vi "main(Test DQMH modules).bak.vi"() -> ()   [LabVIEW 2018, in "Application.lvlib"] (continued)
            frame 0 {
              n828 = Initialize Array(FALSE, 6 ("dimension size")) -> (w2002:bool[])
              n829 = call "MB01_eMICs.vi"("Array"=w2002) -> ("error out"=w2005:errorcluster)  [unwired: 10 in]
            }
            frame 1 {
              n830 = call "demux1-10_chan0.vi"() -> ("error out"=w2006:errorcluster)  [unwired: 11 in]
            }
            frame 2 {
              n831 = call "SC enable OFF.vi"() -> ("error out"=w2007:errorcluster)  [unwired: 11 in]
            }
            frame 3 {
              n832 = call "mux10-1_chan0.vi"() -> ("error out"=w2008:errorcluster)  [unwired: 11 in]
            }
            frame 4 {
              n833 = call "mux6-1_chan0.vi"() -> ("error out"=w2009:errorcluster)  [unwired: 11 in]
            }
            frame 5.., Default {
            }
          }
          n834 = Wait (ms)(milliseconds to wait=u32 70) -> ()  [unwired: 1 out]
        }
        n835 = Merge Errors(w1985, w1989) -> (w1982:errorcluster)
      }
      frame "MEAS.AllRelaysOFF2" {
        n836 = disable-structure shown="LOGGING==TRUE" {
          disable-tunnel: w2013 -> [w2027 _]
          frame condition #0 (active) {
            n837 = Empty String/Path?(string/path=w2027) -> (empty?=w2030:bool)
            n838 = Select(t="Quece timeout", s=w2030, f=w2027) -> (s? t:f=w2026:string)
            n839 = call "string log (SubVI).vi"("Enum"=enum16{"Init", "Log", "Read"}."Log", "state Name"=w2026) -> ()  [unwired: 8 in, 2 out]
          }
          frame condition #1 {
          }
        }
        n840 = flat-sequence {
          tunnel: [w2025] -> w2011
          frame #0 {
            n841 = Initialize Array(FALSE, 6 ("dimension size")) -> (w2024:bool[])
            n842 = call "MB01_eMICs.vi"("Array"=w2024) -> ("error out"=w2025:errorcluster)  [unwired: 10 in]
            n843 = Wait (ms)(milliseconds to wait=u32 70) -> ()  [unwired: 1 out]
          }
        }
        n844 = Merge Errors(w2014, w2011) -> (w2010:errorcluster)
      }
      frame "MEAS.Read TRIGGER" {
        w2042 = T10 {"new board?"=TRUE, "new trigger"=TRUE, "last trigger"=TRUE}  # trigger infor
        # "JIG locked - rising-edge happens"
        n845 = disable-structure shown="LOGGING==TRUE" {
          disable-tunnel: w2046 -> [w2060 _]
          frame condition #0 (active) {
            n846 = Empty String/Path?(string/path=w2060) -> (empty?=w2063:bool)
            n847 = Select(t="Quece timeout", s=w2063, f=w2060) -> (s? t:f=w2059:string)
            n848 = call "string log (SubVI).vi"("Enum"=enum16{"Init", "Log", "Read"}."Log", "state Name"=w2059) -> ()  [unwired: 8 in, 2 out]
          }
          frame condition #1 {
          }
        }
        n849 = call "Read JIG trigger.vi"() -> ("error out"=w2050:errorcluster, "Trigger?"=w2032:bool)  [unwired: 9 in, 1 out]
        "trigger Value" <- w2032
        n850 = feedback-in #3(w2032) -> ()
        n851 = feedback #3(FALSE) -> (w2039:bool)
        n852 = Greater?(x=w2032, y=w2039) -> (0:w2034:bool)
        n853 = Bundle By Name(cluster=w2042, "new board?"=w2034, "new trigger"=w2032, "last trigger"=w2039) -> (w2041:T10)
        n854 = local read "Auto/Man"() -> (w2031:bool)
        n855 = Select(t=-1, s=w2034, f=w2036) -> (s? t:f=w2037:i32)
        n856 = local write "New board?"(w2034) -> ()
        n857 = local write "new Trigger?"(w2032) -> ()
        n858 = local write "last Trigger?"(w2039) -> ()
        n859 = And(x=w2031, y=w2034) -> (x .and. y?=w2033:bool)
        n860 = Merge Errors(w2049, w2050) -> (w2047:errorcluster)
        n861 = case shown="True" w2033 {
          tunnel: w2043 -> [_ w2058]
          tunnel: w2041 -> [_ w2057]
          tunnel: [_ w2056] -> w2040
          frame False {
          }
          frame True {
            n862 = Generate User Event(user event=w2058, event data cluster=w2057) -> (error out=w2056:errorcluster)  [unwired: 2 in, 1 out]
          }
        }
        n863 = Merge Errors(w2047, w2040) -> (w2044:errorcluster)
        n864 = flat-sequence {
          tunnel: [w2064] -> w2048
          tunnel: w2044 -> [w2064]
          frame #0 {
            n865 = Wait (ms)(milliseconds to wait=u32 10) -> ()  [unwired: 1 out]
          }
        }
      }
      frame "MEAS.Sel Input Current" {
        n866 = disable-structure shown="LOGGING==TRUE" {
          disable-tunnel: w2067 -> [w2082 _]
          frame condition #0 (active) {
            n867 = Empty String/Path?(string/path=w2082) -> (empty?=w2085:bool)
            n868 = Select(t="Quece timeout", s=w2085, f=w2082) -> (s? t:f=w2081:string)
            n869 = call "string log (SubVI).vi"("Enum"=enum16{"Init", "Log", "Read"}."Log", "state Name"=w2081) -> ()  [unwired: 8 in, 2 out]
          }
          frame condition #1 {
          }
        }
        n870 = Variant To Data(type=enum16{"DMM I (0.5)", "DMM I (12)"}."DMM I (0.5)" ("mux2-1(DMM I) encode"), Variant=w2075) -> (data=w2074:enum16{"DMM I (0.5)", "DMM I (12)"})  [unwired: 1 in, 1 out]
        n871 = call "DMM I 0.5_10.vi"("mux2-1(DMM I) encode"=w2074) -> ("error out"=w2077:errorcluster)  [unwired: 10 in]
        n872 = Merge Errors(w2070, w2077) -> (w2068:errorcluster)
        n873 = flat-sequence {
          tunnel: [w2086] -> w2069
          tunnel: w2068 -> [w2086]
          frame #0 {
            n874 = Wait (ms)(milliseconds to wait=u32 70) -> ()  [unwired: 1 out]
          }
        }
      }
      frame "MEAS.Read Optos" {
        n875 = disable-structure shown="LOGGING==TRUE" {
          disable-tunnel: w2091 -> [w2116 _]
          frame condition #0 (active) {
            n876 = Empty String/Path?(string/path=w2116) -> (empty?=w2119:bool)
            n877 = Select(t="Quece timeout", s=w2119, f=w2116) -> (s? t:f=w2115:string)
            n878 = call "string log (SubVI).vi"("Enum"=enum16{"Init", "Log", "Read"}."Log", "state Name"=w2115) -> ()  [unwired: 8 in, 2 out]
          }
          frame condition #1 {
          }
        }
        n879 = flat-sequence {
          tunnel: [w2105] -> w2089
          frame #0 {
            n880 = disable-structure shown="Enabled" {
              frame Enabled {
                n881 = Wait (ms)(milliseconds to wait=u32 100) -> ()  [unwired: 1 out]
              }
              frame Disabled {
              }
            }
            n882 = Initialize Array(FALSE, 6 ("dimension size"), 10 ("dimension size")) -> (w2100:bool[][])
            n883 = local write "Short DRV"(w2100) -> ()
          }
          frame #1 {
            n884 = call "inst.Optos.vi"() -> ("error out"=w2114:errorcluster, "Optos"=w2112:bool[])  [unwired: 9 in, 1 out]
            n885 = Reshape Array(w2112, 10 ("dimension size"), 6 ("dimension size")) -> (w2110:bool[][])
            n886 = To Variant(anything=w2112) -> (Variant=w2113:variant)
            n887 = Transpose 2D Array(2D array=w2110) -> (transposed array=→"Short DRV":bool[][])
            n888 = call "FGV Driver Data.vi"("Mode"=DUT_data_Mode."Short Circuits", "error in (no error)"=w2114, "FGV enum(Read)"=FGV_DRV_data."Write" ("FGV DRV data enum"), "data"=w2113) -> ("error out"=w2105:errorcluster)  [unwired: 4 in, 3 out]
          }
        }
        n889 = Merge Errors(w2090, w2089) -> (w2092:errorcluster)
        n890 = flat-sequence {
          tunnel: [w2120] -> w2093
          tunnel: w2092 -> [w2120]
          frame #0 {
            n891 = Wait (ms)(milliseconds to wait=u32 70) -> ()  [unwired: 1 out]
          }
        }
      }
      frame "MEAS.Reset JIG" {
        n892 = disable-structure shown="LOGGING==TRUE" {
          disable-tunnel: w2126 -> [w2136 _]
          frame condition #0 (active) {
            n893 = Empty String/Path?(string/path=w2136) -> (empty?=w2139:bool)
            n894 = Select(t="Quece timeout", s=w2139, f=w2136) -> (s? t:f=w2135:string)
            n895 = call "string log (SubVI).vi"("Enum"=enum16{"Init", "Log", "Read"}."Log", "state Name"=w2135) -> ()  [unwired: 8 in, 2 out]
          }
          frame condition #1 {
          }
        }
        n896 = disable-structure shown="Disabled" {
          disable-tunnel: w2124 -> [w2134 _]
          frame Disabled {
            n897 = call "reset DRV UI (SubVI).vi"("Ref  in"=w2134) -> ()  [unwired: 9 in, 2 out]
          }
          frame Enabled {
          }
        }
        n898 = call "JIG Reset.vi"() -> ("error out"=w2131:errorcluster)  [unwired: 11 in]
        n899 = Merge Errors(w2127, w2131) -> (w2122:errorcluster)
      }
      frame "MEAS.Turn+5V" {
        n900 = disable-structure shown="LOGGING==TRUE" {
          disable-tunnel: w2142 -> [w2158 _]
          frame condition #0 (active) {
            n901 = Empty String/Path?(string/path=w2158) -> (empty?=w2161:bool)
            n902 = Select(t="Quece timeout", s=w2161, f=w2158) -> (s? t:f=w2157:string)
            n903 = call "string log (SubVI).vi"("Enum"=enum16{"Init", "Log", "Read"}."Log", "state Name"=w2157) -> ()  [unwired: 8 in, 2 out]
          }
          frame condition #1 {
          }
        }
        n904 = Variant To Data(type=TRUE, Variant=w2151) -> (data=w2141:bool)  [unwired: 1 in, 1 out]
        n905 = case shown="True" w2141 {
          tunnel: [w2155 w2156] -> w2148
          frame False {
            n906 = call "SC enable OFF.vi"() -> ("error out"=w2155:errorcluster)  [unwired: 11 in]
          }
          frame True {
            n907 = call "SC enable ON.vi"() -> ("error out"=w2156:errorcluster)  [unwired: 11 in]
          }
        }
        n908 = Merge Errors(w2143, w2148) -> (w2144:errorcluster)
        n909 = flat-sequence {
          tunnel: w2144 -> [w2162]
          tunnel: [w2162] -> w2147
          frame #0 {
            n910 = Wait (ms)(milliseconds to wait=u32 2000) -> ()  [unwired: 1 out]
          }
        }
      }
      frame "MEAS.demux1-10" {
        n911 = disable-structure shown="LOGGING==TRUE" {
          disable-tunnel: w2167 -> [w2196 _]
          frame condition #0 (active) {
            n912 = Empty String/Path?(string/path=w2196) -> (empty?=w2199:bool)
            n913 = Select(t="Quece timeout", s=w2199, f=w2196) -> (s? t:f=w2195:string)
            n914 = call "string log (SubVI).vi"("Enum"=enum16{"Init", "Log", "Read"}."Log", "state Name"=w2195) -> ()  [unwired: 8 in, 2 out]
          }
          frame condition #1 {
          }
        }
        n915 = Variant To Data(type=T6."demux1_10_channel0" ("demux1_10(x6)_encode"), Variant=w2175) -> (data=w2166:T6)  [unwired: 1 in, 1 out]
        n916 = case shown="\"demux1_10_channel1\"" w2166 {
          tunnel: [w2184 w2185 w2186 w2187 w2188 w2189 w2190 w2191 w2192 w2193 w2194] -> w2165
          frame "demux1_10_channel0", Default {
            n917 = call "demux1-10_chan0.vi"() -> ("error out"=w2184:errorcluster)  [unwired: 11 in]
          }
          frame "demux1_10_channel1" {
            n918 = call "demux1-10_chan1.vi"() -> ("error out"=w2185:errorcluster)  [unwired: 11 in]
          }
          frame "demux1_10_channel2" {
            n919 = call "demux1-10_chan2.vi"() -> ("error out"=w2186:errorcluster)  [unwired: 11 in]
          }
          frame "demux1_10_channel3" {
            n920 = call "demux1-10_chan3.vi"() -> ("error out"=w2187:errorcluster)  [unwired: 11 in]
          }
          frame "demux1_10_channel4" {
            n921 = call "demux1-10_chan4.vi"() -> ("error out"=w2188:errorcluster)  [unwired: 11 in]
          }
          frame "demux1_10_channel5" {
            n922 = call "demux1-10_chan5.vi"() -> ("error out"=w2189:errorcluster)  [unwired: 11 in]
          }
          frame "demux1_10_channel6" {
            n923 = call "demux1-10_chan6.vi"() -> ("error out"=w2190:errorcluster)  [unwired: 11 in]
          }
          frame "demux1_10_channel7" {
            n924 = call "demux1-10_chan7.vi"() -> ("error out"=w2191:errorcluster)  [unwired: 11 in]
          }
          frame "demux1_10_channel8" {
            n925 = call "demux1-10_chan8.vi"() -> ("error out"=w2192:errorcluster)  [unwired: 11 in]
          }
          frame "demux1_10_channel9" {
            n926 = call "demux1-10_chan9.vi"() -> ("error out"=w2193:errorcluster)  [unwired: 11 in]
          }
          frame "demux1_10_channel10" {
            n927 = call "demux1-10_chan10.vi"() -> ("error out"=w2194:errorcluster)  [unwired: 11 in]
          }
        }
        n928 = Merge Errors(w2168, w2165) -> (w2169:errorcluster)
        n929 = disable-structure shown="Enabled" {
          disable-tunnel: [w2180 w2183] -> w2170
          disable-tunnel: w2169 -> [w2179 w2183]
          frame Enabled {
            n930 = flat-sequence {
              tunnel: [w2181] -> w2180
              tunnel: w2179 -> [w2181]
              frame #0 {
                n931 = Wait (ms)(milliseconds to wait="1-10delay") -> ()  [unwired: 1 out]
              }
            }
          }
          frame Disabled {
          }
        }
      }
      frame "MEAS.eMIC" {
        # "eliminated shorted Circuits"
        n932 = disable-structure shown="LOGGING==TRUE" {
          disable-tunnel: w2202 -> [w2228 _]
          frame condition #0 (active) {
            n933 = Empty String/Path?(string/path=w2228) -> (empty?=w2231:bool)
            n934 = Select(t="Quece timeout", s=w2231, f=w2228) -> (s? t:f=w2227:string)
            n935 = call "string log (SubVI).vi"("Enum"=enum16{"Init", "Log", "Read"}."Log", "state Name"=w2227) -> ()  [unwired: 8 in, 2 out]
          }
          frame condition #1 {
          }
        }
        n936 = call "FGV Driver Data.vi"("DUT channel (1-11)"=w2204, "FGV enum(Read)"=FGV_DRV_data."Read" ("FGV DRV data enum")) -> ("Short Circuits?"=w2213:bool[])  [unwired: 6 in, 3 out]
        n937 = Variant To Data(type=bool[] [], Variant=w2218) -> (data=w2211:bool[])  [unwired: 1 in, 1 out]
        n938 = Not(x=w2213) -> (.not. x?=w2212:bool[])
        n939 = And(x=w2212, y=w2211) -> (x .and. y?=w2210:bool[])
        n940 = call "MB01_eMICs.vi"("Array"=w2210) -> ("error out"=w2208:errorcluster)  [unwired: 10 in]
        n941 = call "FGV wait for 6 eMICs.vi"("Enum"=enum16{"Init", "count"}."Init", "error in (no error)"=w2208) -> ("error out"=w2200:errorcluster, "wait done"=w2209:bool)  [unwired: 7 in, 1 out]
        n942 = Merge Errors(w2203, w2200) -> (w2205:errorcluster)
        n943 = local write "AC  Completed"(w2209) -> ()
        n944 = disable-structure shown="Enabled" {
          disable-tunnel: [w2223 w2226] -> w2206
          disable-tunnel: w2205 -> [w2222 w2226]
          frame Enabled {
            n945 = flat-sequence {
              tunnel: [w2225] -> w2223
              tunnel: w2222 -> [w2225]
              frame #0 {
                n946 = Wait (ms)(milliseconds to wait="eMIC delay") -> ()  [unwired: 1 out]
              }
            }
          }
          frame Disabled {
          }
        }
      }
      frame "MEAS.requestAC" {
        n947 = disable-structure shown="LOGGING==TRUE" {
          disable-tunnel: w2235 -> [w2264 _]
          frame condition #0 (active) {
            n948 = Empty String/Path?(string/path=w2264) -> (empty?=w2267:bool)
            n949 = Select(t="Quece timeout", s=w2267, f=w2264) -> (s? t:f=w2263:string)
            n950 = call "string log (SubVI).vi"("Enum"=enum16{"Init", "Log", "Read"}."Log", "state Name"=w2263) -> ()  [unwired: 8 in, 2 out]
          }
          frame condition #1 {
          }
        }
        n951 = Variant To Data(type=-1 ("Module ID"), Variant=w2233) -> (data=w2232:i32)  [unwired: 1 in, 1 out]
        n952 = case shown="0" w2232 {
          selector: w2232 -> [w2252 _]
          tunnel: [w2251 w2256] -> w2239
          frame 1, Default {
            n953 = Quotient & Remainder(x=w2252, y=6) -> (x-y*floor(x/y)=w2248:i32)  [unwired: 1 out]
            n954 = Equal To 0?(x=w2248) -> (x = 0?=w2250:bool)
            n955 = Select(t=6, s=w2250, f=w2248) -> (s? t:f=w2247:i32)
            n956 = call "Read AC parameters.vi"("Module ID"=w2247) -> ("error out"=w2251:errorcluster)  [unwired: 10 in]
          }
          frame 0 {
            n957 = call "FGV wait for 6 eMICs.vi"("Enum"=enum16{"Init", "count"}."Init") -> ("error out"=w2254:errorcluster)  [unwired: 8 in, 2 out]
            n958 = call "Read AC parameters.vi"("error in"=w2254, "Module ID"=-1) -> ("error out"=w2256:errorcluster)  [unwired: 9 in]
          }
        }
        n959 = Merge Errors(w2240, w2239) -> (w2237:errorcluster)
        n960 = disable-structure shown="Enabled" {
          disable-tunnel: [w2259 w2262] -> w2238
          disable-tunnel: w2237 -> [w2258 w2262]
          frame Disabled {
            n961 = flat-sequence {
              tunnel: [w2260] -> w2259
              tunnel: w2258 -> [w2260]
              frame #0 {
                n962 = Wait (ms)(milliseconds to wait=u32 70) -> ()  [unwired: 1 out]
              }
            }
          }
          frame Enabled {
          }
        }
      }
      frame "MEAS.mux6_1" {
        n963 = disable-structure shown="LOGGING==TRUE" {
          disable-tunnel: w2274 -> [w2317 _]
          frame condition #0 (active) {
            n964 = Empty String/Path?(string/path=w2317) -> (empty?=w2320:bool)
            n965 = Select(t="Quece timeout", s=w2320, f=w2317) -> (s? t:f=w2316:string)
            n966 = call "string log (SubVI).vi"("Enum"=enum16{"Init", "Log", "Read"}."Log", "state Name"=w2316) -> ()  [unwired: 8 in, 2 out]
          }
          frame condition #1 {
          }
        }
        n967 = Variant To Data(type=T4."mux6-1_channel0" ("mux6_1(3wires)_encode"), Variant=w2282) -> (data=w2273:T4)  [unwired: 1 in, 1 out]
        n968 = case shown="\"mux6_1_channel6_3\"" w2273 {
          tunnel: [w2291 w2293 w2295 w2297 w2299 w2301 w2303 w2305 w2307 w2309 w2311 w2313 w2315] -> w2272
          tunnel: [w2290 w2292 w2294 w2296 w2298 w2300 w2302 w2304 w2306 w2308 w2310 w2312 w2314] -> w2268
          tunnel: "6_1 delay" -> [_ _ w2294 _ w2298 _ w2302 _ w2306 _ w2310 _ w2314]
          tunnel: "6_1 delay2" -> [w2290 w2292 _ w2296 _ w2300 _ w2304 _ w2308 _ w2312 _]
          frame "mux6-1_channel0", Default {
            n969 = call "mux6-1_chan0.vi"() -> ("error out"=w2291:errorcluster)  [unwired: 11 in]
          }
          frame "mux6-1_channel1_2" {
            n970 = call "mux6-1_chan1_1.vi"() -> ("error out"=w2293:errorcluster)  [unwired: 11 in]
          }
          frame "mux6_1_channel1_3" {
            n971 = call "mux6-1_chan1_2.vi"() -> ("error out"=w2295:errorcluster)  [unwired: 11 in]
          }
          frame "mux6_1_channel2_2" {
            n972 = call "mux6-1_chan2_1.vi"() -> ("error out"=w2297:errorcluster)  [unwired: 11 in]
          }
          frame "mux6_1_channel2_3" {
            n973 = call "mux6-1_chan2_2.vi"() -> ("error out"=w2299:errorcluster)  [unwired: 11 in]
          }
          frame "mux6_1_channel3_2" {
            n974 = call "mux6-1_chan3_1.vi"() -> ("error out"=w2301:errorcluster)  [unwired: 11 in]
          }
          frame "mux6_1_channel3_3" {
            n975 = call "mux6-1_chan3_2.vi"() -> ("error out"=w2303:errorcluster)  [unwired: 11 in]
          }
          frame "mux6_1_channel4_2" {
            n976 = call "mux6-1_chan4_1.vi"() -> ("error out"=w2305:errorcluster)  [unwired: 11 in]
          }
          frame "mux6_1_channel4_3" {
            n977 = call "mux6-1_chan4_2.vi"() -> ("error out"=w2307:errorcluster)  [unwired: 11 in]
          }
          frame "mux6_1_channel5_2" {
            n978 = call "mux6-1_chan5_1.vi"() -> ("error out"=w2309:errorcluster)  [unwired: 11 in]
          }
          frame "mux6_1_channel5_3" {
            n979 = call "mux6-1_chan5_2.vi"() -> ("error out"=w2311:errorcluster)  [unwired: 11 in]
          }
          frame "mux6_1_channel6_2" {
            n980 = call "mux6-1_chan6_1.vi"() -> ("error out"=w2313:errorcluster)  [unwired: 11 in]
          }
          frame "mux6_1_channel6_3" {
            n981 = call "mux6-1_chan6_2.vi"() -> ("error out"=w2315:errorcluster)  [unwired: 11 in]
          }
        }
        n982 = Merge Errors(w2277, w2272) -> (w2275:errorcluster)
        n983 = Wait (ms)(milliseconds to wait=w2268) -> ()  [unwired: 1 out]
        n984 = disable-structure shown="Enabled" {
          disable-tunnel: [w2287 w2289] -> w2276
          disable-tunnel: w2275 -> [w2286 w2289]
          frame Enabled {
            n985 = flat-sequence {
              tunnel: [w2288] -> w2287
              tunnel: w2286 -> [w2288]
              frame #0 {
              }
            }
          }
          frame Disabled {
          }
        }
      }
      frame "MEAS.mux10-1" {
        n986 = disable-structure shown="LOGGING==TRUE" {
          disable-tunnel: w2324 -> [w2353 _]
          frame condition #0 (active) {
            n987 = Empty String/Path?(string/path=w2353) -> (empty?=w2356:bool)
            n988 = Select(t="Quece timeout", s=w2356, f=w2353) -> (s? t:f=w2352:string)
            n989 = call "string log (SubVI).vi"("Enum"=enum16{"Init", "Log", "Read"}."Log", "state Name"=w2352) -> ()  [unwired: 8 in, 2 out]
          }
          frame condition #1 {
          }
        }
        n990 = Variant To Data(type=T5."mux10_1_channel0" ("mux10_1(x6)_encode"), Variant=w2332) -> (data=w2323:T5)  [unwired: 1 in, 1 out]
        n991 = case shown="\"mux10_1_channel1\"" w2323 {
          tunnel: [w2341 w2342 w2343 w2344 w2345 w2346 w2347 w2348 w2349 w2350 w2351] -> w2322
          frame "mux10_1_channel0", Default {
            n992 = call "mux10-1_chan0.vi"() -> ("error out"=w2341:errorcluster)  [unwired: 11 in]
          }
          frame "mux10_1_channel1" {
            n993 = call "mux10-1_chan1.vi"() -> ("error out"=w2342:errorcluster)  [unwired: 11 in]
          }
          frame "mux10_1_channel2" {
            n994 = call "mux10-1_chan2.vi"() -> ("error out"=w2343:errorcluster)  [unwired: 11 in]
          }
          frame "mux10_1_channel3" {
            n995 = call "mux10-1_chan3.vi"() -> ("error out"=w2344:errorcluster)  [unwired: 11 in]
          }
          frame "mux10_1_channel4" {
            n996 = call "mux10-1_chan4.vi"() -> ("error out"=w2345:errorcluster)  [unwired: 11 in]
          }
          frame "mux10_1_channel5" {
            n997 = call "mux10-1_chan5.vi"() -> ("error out"=w2346:errorcluster)  [unwired: 11 in]
          }
          frame "mux10_1_channel6" {
            n998 = call "mux10-1_chan6.vi"() -> ("error out"=w2347:errorcluster)  [unwired: 11 in]
          }
          frame "mux10_1_channel7" {
            n999 = call "mux10-1_chan7.vi"() -> ("error out"=w2348:errorcluster)  [unwired: 11 in]
          }
          frame "mux10_1_channel8" {
            n1000 = call "mux10-1_chan8.vi"() -> ("error out"=w2349:errorcluster)  [unwired: 11 in]
          }
          frame "mux10_1_channel9" {
            n1001 = call "mux10-1_chan9.vi"() -> ("error out"=w2350:errorcluster)  [unwired: 11 in]
          }
          frame "mux10_1_channel10" {
            n1002 = call "mux10-1_chan10.vi"() -> ("error out"=w2351:errorcluster)  [unwired: 11 in]
          }
        }
        n1003 = Merge Errors(w2327, w2322) -> (w2326:errorcluster)
        n1004 = disable-structure shown="Enabled" {
          disable-tunnel: w2326 -> [w2337 w2340]
          disable-tunnel: [w2336 w2340] -> w2325
          frame Enabled {
            n1005 = flat-sequence {
              tunnel: w2337 -> [w2338]
              tunnel: [w2338] -> w2336
              frame #0 {
                n1006 = Wait (ms)(milliseconds to wait="10-1 delay") -> ()  [unwired: 1 out]
              }
            }
          }
          frame Disabled {
          }
        }
      }
      frame "MEAS.DMM dual read" {
        n1007 = disable-structure shown="LOGGING==TRUE" {
          disable-tunnel: w2364 -> [w2390 _]
          frame condition #0 (active) {
            n1008 = Empty String/Path?(string/path=w2390) -> (empty?=w2393:bool)
            n1009 = Select(t="Quece timeout", s=w2393, f=w2390) -> (s? t:f=w2389:string)
            n1010 = call "string log (SubVI).vi"("Enum"=enum16{"Init", "Log", "Read"}."Log", "state Name"=w2389) -> ()  [unwired: 8 in, 2 out]
          }
          frame condition #1 {
          }
        }
        n1011 = call "FGV Driver Data.vi"("DUT index(1-60)"=w2357) -> ("DUT SC"=w2358:bool)  [unwired: 7 in, 3 out]
        n1012 = case shown="False" w2358 {
          tunnel: [w2371 _] -> w2360
          tunnel: w2357 -> [w2372 _]
          frame False {
            n1013 = flat-sequence {
              tunnel: [w2375] -> w2373
              tunnel: w2372 -> [w2375]
              tunnel: w2373 -> [w2378]
              tunnel: [w2377] -> w2371
              frame #0 {
                w2374 = 0.0 ("DCV(Volts)")
                n1014 = disable-structure shown="Enabled" {
                  frame Enabled {
                    n1015 = Wait (ms)(milliseconds to wait=u32 50) -> ()  [unwired: 1 out]
                  }
                  frame Disabled {
                  }
                }
                n1016 = local write "DCV(Volts)"(w2374) -> ()
                n1017 = local write "DCI(mA)"(w2374) -> ()
              }
              frame #1 {
                w2379 = u16 2 items=["1st Display", "2nd Display", "1st & 2nd Display"] ("Sets to Display")
                n1018 = call "Read DCV_DCI.vi"("Sets to Display"=w2379) -> ("error out"=w2382:errorcluster, "DCI"=w2386:dbl, "DCV"=w2385:dbl)  [unwired: 7 in, 1 out]
                "DCI(mA)" <- w2386
                "DCV(Volts)" <- w2385
                n1019 = Build Array(w2385, w2386) -> (w2384:dbl[])
                n1020 = To Variant(anything=w2384) -> (Variant=w2383:variant)
                n1021 = call "FGV Driver Data.vi"("Mode"=DUT_data_Mode."DC parameter", "DUT index(1-60)"=w2378, "error in (no error)"=w2382, "FGV enum(Read)"=FGV_DRV_data."Write" ("FGV DRV data enum"), "data"=w2383) -> ("error out"=w2377:errorcluster)  [unwired: 3 in, 3 out]
              }
            }
          }
          frame True {
          }
        }
        n1022 = Merge Errors(w2365, w2360) -> (w2362:errorcluster)
        n1023 = flat-sequence {
          tunnel: [w2388] -> w2363
          tunnel: w2362 -> [w2388]
          frame #0 {
            n1024 = Wait (ms)(milliseconds to wait="DMM delay") -> ()  [unwired: 1 out]
          }
        }
      }
      frame "Test Shorted Circuits" {
        w2400 = T25 {"command"="", "Data"=variant} ("Variant")
        n1025 = disable-structure shown="LOGGING==TRUE" {
          disable-tunnel: w2409 -> [w2429 _]
          frame condition #0 (active) {
            n1026 = Empty String/Path?(string/path=w2429) -> (empty?=w2432:bool)
            n1027 = Select(t="Quece timeout", s=w2432, f=w2429) -> (s? t:f=w2428:string)
            n1028 = call "string log (SubVI).vi"("Enum"=enum16{"Init", "Log", "Read"}."Log", "state Name"=w2428) -> ()  [unwired: 8 in, 2 out]
          }
          frame condition #1 {
          }
        }
        n1029 = To Variant(anything=TRUE) -> (Variant=w2419:variant)
        n1030 = To Variant(anything=FALSE) -> (Variant=w2404:variant)
        n1031 = Bundle By Name(cluster=w2400, "command"="MEAS.AllRelaysOFF") -> (w2421:T25)
        n1032 = Bundle By Name(cluster=w2400, "command"="MEAS.Turn+5V", "Data"=w2419) -> (w2420:T25)
        n1033 = Bundle By Name(cluster=w2400, "command"="MEAS.Read Optos") -> (w2417:T25)
        n1034 = Bundle By Name(cluster=w2400, "command"="MEAS.Turn+5V", "Data"=w2404) -> (w2408:T25)
        n1035 = Bundle By Name(cluster=w2400, "command"="Apps.UI Update SC") -> (w2398:T25)
        n1036 = Build Array(w2421, w2420, w2417, w2408, w2398) -> (w2410:T25[])
        n1037 = Reverse 1D Array(array=w2410) -> (reversed array=w2411:T25[])
        n1038 = for {
          tunnel: w2411 -> [w2436] mode=indexing
          tunnel: w2415 -> [w2438]
          tunnel: [w2437] -> w2402 mode=indexing
          n1039 = Unbundle By Name(w2436) -> ("command"=w2435:string, "Data"=w2434:variant)
          n1040 = call "App enquece.vi"("Priority Enquece"=TRUE, "command data"=w2434, "command"=w2435, "queue in"=w2438) -> ("error out"=w2437:errorcluster)  [unwired: 6 in, 1 out]
        }
        n1041 = call "reset DRV UI (SubVI).vi"("Ref  in"=w2414) -> ("error out"=w2395:errorcluster)  [unwired: 9 in, 1 out]
        n1042 = call "FGV Driver Data.vi"("error in (no error)"=w2395, "FGV enum(Read)"=FGV_DRV_data."Init" ("FGV DRV data enum")) -> ("error out"=w2394:errorcluster)  [unwired: 6 in, 3 out]
        n1043 = Merge Errors(w2403, w2402) -> (w2407:errorcluster)
        n1044 = Merge Errors(w2407, w2394) -> (w2397:errorcluster)
      }
      frame "Test Channel 1" {
        w2468 = 1  # DUT channel (1-11)
        w2469 = T11 {"command"="", "command data"=variant} ("element")
        n1045 = disable-structure shown="LOGGING==TRUE" {
          disable-tunnel: w2464 -> [w2499 _]
          frame condition #0 (active) {
            n1046 = Empty String/Path?(string/path=w2499) -> (empty?=w2502:bool)
            n1047 = Select(t="Quece timeout", s=w2502, f=w2499) -> (s? t:f=w2498:string)
            n1048 = call "string log (SubVI).vi"("Enum"=enum16{"Init", "Log", "Read"}."Log", "state Name"=w2498) -> ()  [unwired: 8 in, 2 out]
          }
          frame condition #1 {
          }
        }
        n1049 = Build Array("Apps.UI Update", "MEAS.AllRelaysOFF2", "Apps.WaitForEvent") -> (w2448:string[])
        n1050 = for {
          tunnel: [w2489] -> w2450 mode=indexing
          shift-right: [w2488] -> w2449
          shift-left: w2451 -> [w2491]
          tunnel: w2448 -> [w2487] mode=indexing
          n1051 = call "App enquece.vi"("Priority Enquece"=TRUE, "command"=w2487, "queue in"=w2491) -> ("error out"=w2489:errorcluster, "Queue out"=w2488:refnum<queue>)  [unwired: 7 in]
        }
        n1052 = Build Array("Test DRV 1", "Test DRV 2", "Test DRV 3", "Test DRV 4", "Test DRV 5", "Test DRV 6", "MEAS.requestAC") -> (w2461:string[])
        n1053 = Merge Errors(w2450) -> (w2445:errorcluster)
        n1054 = Reverse 1D Array(array=w2461) -> (reversed array=w2462:string[])
        n1055 = for {
          tunnel: w2462 -> [w2496] mode=indexing
          tunnel: [w2495] -> w2455 mode=indexing
          shift-right: [w2494] -> w2456
          shift-left: w2449 -> [w2497]
          tunnel: w2445 -> [w2493]
          n1056 = call "App enquece.vi"("Priority Enquece"=TRUE, "error in (no error)"=w2493, "command"=w2496, "queue in"=w2497) -> ("error out"=w2495:errorcluster, "Queue out"=w2494:refnum<queue>)  [unwired: 6 in]
        }
        n1057 = Initialize Array(TRUE, 6 ("dimension size")) -> (w2472:bool[])
        n1058 = To Variant(anything=w2472) -> (Variant=w2471:variant)
        n1059 = To Variant(anything=T6."demux1_10_channel1" ("demux1_10(x6)_encode")) -> (Variant=w2478:variant)
        n1060 = To Variant(anything=T5."mux10_1_channel1" ("mux10_1(x6)_encode")) -> (Variant=w2482:variant)
        n1061 = Bundle By Name(cluster=w2469, "command"="MEAS.mux10-1", "command data"=w2482) -> (w2477:T11)
        n1062 = Bundle By Name(cluster=w2469, "command"="MEAS.demux1-10", "command data"=w2478) -> (w2476:T11)
        n1063 = Bundle By Name(cluster=w2469, "command"="MEAS.eMIC", "command data"=w2471) -> (w2470:T11)
        n1064 = Build Array(w2477, w2476, w2470) -> (w2453:T11[])
        n1065 = Merge Errors(w2455) -> (w2454:errorcluster)
        n1066 = Reverse 1D Array(array=w2453) -> (reversed array=w2452:T11[])
        n1067 = for {
          tunnel: w2452 -> [w2508] mode=indexing
          tunnel: [w2505] -> w2463 mode=indexing
          tunnel: w2454 -> [w2504]
          tunnel: w2456 -> [w2509]
          n1068 = Unbundle By Name(w2508) -> ("command"=w2507:string, "command data"=w2506:variant)
          n1069 = call "App enquece.vi"("Priority Enquece"=TRUE, "error in (no error)"=w2504, "command data"=w2506, "command"=w2507, "queue in"=w2509) -> ("error out"=w2505:errorcluster)  [unwired: 5 in, 1 out]
        }
        n1070 = Merge Errors(w2466, w2463) -> (w2467:errorcluster)
      }
      frame "Test Channel 2" {
        w2541 = 2  # DUT channel (1-11)
        w2542 = T11 {"command"="", "command data"=variant} ("element")
        n1071 = disable-structure shown="LOGGING==TRUE" {
          disable-tunnel: w2536 -> [w2570 _]
          frame condition #0 (active) {
            n1072 = Empty String/Path?(string/path=w2570) -> (empty?=w2573:bool)
            n1073 = Select(t="Quece timeout", s=w2573, f=w2570) -> (s? t:f=w2569:string)
            n1074 = call "string log (SubVI).vi"("Enum"=enum16{"Init", "Log", "Read"}."Log", "state Name"=w2569) -> ()  [unwired: 8 in, 2 out]
          }
          frame condition #1 {
          }
        }
        n1075 = Build Array("Apps.UI Update", "MEAS.AllRelaysOFF2", "Apps.WaitForEvent") -> (w2515:string[])
        n1076 = for {
          tunnel: [w2561] -> w2526 mode=indexing
          shift-right: [w2562] -> w2528
          shift-left: w2521 -> [w2560]
          tunnel: w2515 -> [w2558] mode=indexing
          n1077 = call "App enquece.vi"("Priority Enquece"=TRUE, "command"=w2558, "queue in"=w2560) -> ("error out"=w2561:errorcluster, "Queue out"=w2562:refnum<queue>)  [unwired: 7 in]
        }
        n1078 = Merge Errors(w2526) -> (w2518:errorcluster)
        n1079 = Build Array("Test DRV 7", "Test DRV 8", "Test DRV 9", "Test DRV 10", "Test DRV 11", "Test DRV 12", "MEAS.requestAC") -> (w2533:string[])
        n1080 = Reverse 1D Array(array=w2533) -> (reversed array=w2534:string[])
        n1081 = for {
          tunnel: w2534 -> [w2563] mode=indexing
          tunnel: [w2567] -> w2525 mode=indexing
          shift-right: [w2566] -> w2527
          shift-left: w2528 -> [w2568]
          tunnel: w2518 -> [w2565]
          n1082 = call "App enquece.vi"("Priority Enquece"=TRUE, "error in (no error)"=w2565, "command"=w2563, "queue in"=w2568) -> ("error out"=w2567:errorcluster, "Queue out"=w2566:refnum<queue>)  [unwired: 6 in]
        }
        n1083 = Initialize Array(TRUE, 6 ("dimension size")) -> (w2545:bool[])
        n1084 = To Variant(anything=T5."mux10_1_channel2" ("mux10_1(x6)_encode")) -> (Variant=w2553:variant)
        n1085 = To Variant(anything=T6."demux1_10_channel2" ("demux1_10(x6)_encode")) -> (Variant=w2550:variant)
        n1086 = To Variant(anything=w2545) -> (Variant=w2544:variant)
        n1087 = Bundle By Name(cluster=w2542, "command"="MEAS.mux10-1", "command data"=w2553) -> (w2549:T11)
        n1088 = Bundle By Name(cluster=w2542, "command"="MEAS.demux1-10", "command data"=w2550) -> (w2548:T11)
        n1089 = Bundle By Name(cluster=w2542, "command"="MEAS.eMIC", "command data"=w2544) -> (w2543:T11)
        n1090 = Merge Errors(w2525) -> (w2524:errorcluster)
        n1091 = Build Array(w2549, w2548, w2543) -> (w2523:T11[])
        n1092 = Reverse 1D Array(array=w2523) -> (reversed array=w2522:T11[])
        n1093 = for {
          tunnel: w2522 -> [w2579] mode=indexing
          tunnel: [w2576] -> w2535 mode=indexing
          tunnel: w2524 -> [w2575]
          tunnel: w2527 -> [w2580]
          n1094 = Unbundle By Name(w2579) -> ("command"=w2578:string, "command data"=w2577:variant)
          n1095 = call "App enquece.vi"("Priority Enquece"=TRUE, "error in (no error)"=w2575, "command data"=w2577, "command"=w2578, "queue in"=w2580) -> ("error out"=w2576:errorcluster)  [unwired: 5 in, 1 out]
        }
        n1096 = Merge Errors(w2538, w2535) -> (w2539:errorcluster)
      }
      frame "Test Channel 3" {
        w2611 = 3  # DUT channel (1-11)
        w2612 = T11 {"command"="", "command data"=variant} ("element")
        n1097 = disable-structure shown="LOGGING==TRUE" {
          disable-tunnel: w2606 -> [w2641 _]
          frame condition #0 (active) {
            n1098 = Empty String/Path?(string/path=w2641) -> (empty?=w2644:bool)
            n1099 = Select(t="Quece timeout", s=w2644, f=w2641) -> (s? t:f=w2640:string)
            n1100 = call "string log (SubVI).vi"("Enum"=enum16{"Init", "Log", "Read"}."Log", "state Name"=w2640) -> ()  [unwired: 8 in, 2 out]
          }
          frame condition #1 {
          }
        }
        n1101 = Build Array("Apps.UI Update", "MEAS.AllRelaysOFF2", "Apps.WaitForEvent") -> (w2589:string[])
        n1102 = for {
          tunnel: [w2631] -> w2596 mode=indexing
          shift-right: [w2632] -> w2598
          shift-left: w2592 -> [w2630]
          tunnel: w2589 -> [w2629] mode=indexing
          n1103 = call "App enquece.vi"("Priority Enquece"=TRUE, "command"=w2629, "queue in"=w2630) -> ("error out"=w2631:errorcluster, "Queue out"=w2632:refnum<queue>)  [unwired: 7 in]
        }
        n1104 = Merge Errors(w2596) -> (w2588:errorcluster)
        n1105 = Build Array("Test DRV 13", "Test DRV 14", "Test DRV 15", "Test DRV 16", "Test DRV 17", "Test DRV 18", "MEAS.requestAC") -> (w2603:string[])
        n1106 = Reverse 1D Array(array=w2603) -> (reversed array=w2604:string[])
        n1107 = for {
          tunnel: w2604 -> [w2638] mode=indexing
          tunnel: [w2637] -> w2583 mode=indexing
          shift-right: [w2636] -> w2597
          shift-left: w2598 -> [w2639]
          tunnel: w2588 -> [w2635]
          n1108 = call "App enquece.vi"("Priority Enquece"=TRUE, "error in (no error)"=w2635, "command"=w2638, "queue in"=w2639) -> ("error out"=w2637:errorcluster, "Queue out"=w2636:refnum<queue>)  [unwired: 6 in]
        }
        n1109 = Merge Errors(w2583) -> (w2595:errorcluster)
        n1110 = Initialize Array(TRUE, 6 ("dimension size")) -> (w2615:bool[])
        n1111 = To Variant(anything=T5."mux10_1_channel3" ("mux10_1(x6)_encode")) -> (Variant=w2624:variant)
        n1112 = To Variant(anything=T6."demux1_10_channel3" ("demux1_10(x6)_encode")) -> (Variant=w2620:variant)
        n1113 = To Variant(anything=w2615) -> (Variant=w2614:variant)
        n1114 = Bundle By Name(cluster=w2612, "command"="MEAS.mux10-1", "command data"=w2624) -> (w2619:T11)
        n1115 = Bundle By Name(cluster=w2612, "command"="MEAS.demux1-10", "command data"=w2620) -> (w2618:T11)
        n1116 = Bundle By Name(cluster=w2612, "command"="MEAS.eMIC", "command data"=w2614) -> (w2613:T11)
        n1117 = Build Array(w2619, w2618, w2613) -> (w2594:T11[])
        n1118 = Reverse 1D Array(array=w2594) -> (reversed array=w2593:T11[])
        n1119 = for {
          tunnel: w2593 -> [w2650] mode=indexing
          tunnel: [w2647] -> w2605 mode=indexing
          tunnel: w2595 -> [w2646]
          tunnel: w2597 -> [w2651]
          n1120 = Unbundle By Name(w2650) -> ("command"=w2649:string, "command data"=w2648:variant)
          n1121 = call "App enquece.vi"("Priority Enquece"=TRUE, "error in (no error)"=w2646, "command data"=w2648, "command"=w2649, "queue in"=w2651) -> ("error out"=w2647:errorcluster)  [unwired: 5 in, 1 out]
        }
        n1122 = Merge Errors(w2608, w2605) -> (w2609:errorcluster)
      }
      frame "Test Channel 4" {
        w2682 = 4  # DUT channel (1-11)
        w2683 = T11 {"command"="", "command data"=variant} ("element")
        n1123 = disable-structure shown="LOGGING==TRUE" {
          disable-tunnel: w2677 -> [w2712 _]
          frame condition #0 (active) {
            n1124 = Empty String/Path?(string/path=w2712) -> (empty?=w2715:bool)
            n1125 = Select(t="Quece timeout", s=w2715, f=w2712) -> (s? t:f=w2711:string)
            n1126 = call "string log (SubVI).vi"("Enum"=enum16{"Init", "Log", "Read"}."Log", "state Name"=w2711) -> ()  [unwired: 8 in, 2 out]
          }
          frame condition #1 {
          }
        }
        n1127 = Build Array("Apps.UI Update", "MEAS.AllRelaysOFF2", "Apps.WaitForEvent") -> (w2659:string[])
        n1128 = for {
          tunnel: [w2702] -> w2667 mode=indexing
          shift-right: [w2703] -> w2669
          shift-left: w2662 -> [w2701]
          tunnel: w2659 -> [w2700] mode=indexing
          n1129 = call "App enquece.vi"("Priority Enquece"=TRUE, "command"=w2700, "queue in"=w2701) -> ("error out"=w2702:errorcluster, "Queue out"=w2703:refnum<queue>)  [unwired: 7 in]
        }
        n1130 = Merge Errors(w2667) -> (w2658:errorcluster)
        n1131 = Build Array("Test DRV 19", "Test DRV 20", "Test DRV 21", "Test DRV 22", "Test DRV 23", "Test DRV 24", "MEAS.requestAC") -> (w2674:string[])
        n1132 = Reverse 1D Array(array=w2674) -> (reversed array=w2675:string[])
        n1133 = for {
          tunnel: w2675 -> [w2709] mode=indexing
          tunnel: [w2708] -> w2666 mode=indexing
          shift-right: [w2707] -> w2668
          shift-left: w2669 -> [w2710]
          tunnel: w2658 -> [w2706]
          n1134 = call "App enquece.vi"("Priority Enquece"=TRUE, "error in (no error)"=w2706, "command"=w2709, "queue in"=w2710) -> ("error out"=w2708:errorcluster, "Queue out"=w2707:refnum<queue>)  [unwired: 6 in]
        }
        n1135 = Merge Errors(w2666) -> (w2665:errorcluster)
        n1136 = Initialize Array(TRUE, 6 ("dimension size")) -> (w2686:bool[])
        n1137 = To Variant(anything=T5."mux10_1_channel4" ("mux10_1(x6)_encode")) -> (Variant=w2695:variant)
        n1138 = To Variant(anything=T6."demux1_10_channel4" ("demux1_10(x6)_encode")) -> (Variant=w2691:variant)
        n1139 = To Variant(anything=w2686) -> (Variant=w2685:variant)
        n1140 = Bundle By Name(cluster=w2683, "command"="MEAS.mux10-1", "command data"=w2695) -> (w2690:T11)
        n1141 = Bundle By Name(cluster=w2683, "command"="MEAS.demux1-10", "command data"=w2691) -> (w2689:T11)
        n1142 = Bundle By Name(cluster=w2683, "command"="MEAS.eMIC", "command data"=w2685) -> (w2684:T11)
        n1143 = Build Array(w2690, w2689, w2684) -> (w2664:T11[])
        n1144 = Reverse 1D Array(array=w2664) -> (reversed array=w2663:T11[])
        n1145 = for {
          tunnel: w2663 -> [w2721] mode=indexing
          tunnel: [w2718] -> w2676 mode=indexing
          tunnel: w2665 -> [w2717]
          tunnel: w2668 -> [w2722]
          n1146 = Unbundle By Name(w2721) -> ("command"=w2720:string, "command data"=w2719:variant)
          n1147 = call "App enquece.vi"("Priority Enquece"=TRUE, "error in (no error)"=w2717, "command data"=w2719, "command"=w2720, "queue in"=w2722) -> ("error out"=w2718:errorcluster)  [unwired: 5 in, 1 out]
        }
        n1148 = Merge Errors(w2679, w2676) -> (w2680:errorcluster)
      }
      frame "Test Channel 5" {
        w2753 = 5  # DUT channel (1-11)
        w2754 = T11 {"command"="", "command data"=variant} ("element")
        n1149 = disable-structure shown="LOGGING==TRUE" {
          disable-tunnel: w2748 -> [w2783 _]
          frame condition #0 (active) {
            n1150 = Empty String/Path?(string/path=w2783) -> (empty?=w2786:bool)
            n1151 = Select(t="Quece timeout", s=w2786, f=w2783) -> (s? t:f=w2782:string)
            n1152 = call "string log (SubVI).vi"("Enum"=enum16{"Init", "Log", "Read"}."Log", "state Name"=w2782) -> ()  [unwired: 8 in, 2 out]
          }
          frame condition #1 {
          }
        }
        n1153 = Build Array("Apps.UI Update", "MEAS.AllRelaysOFF2", "Apps.WaitForEvent") -> (w2731:string[])
        n1154 = for {
          tunnel: [w2773] -> w2739 mode=indexing
          shift-right: [w2774] -> w2740
          shift-left: w2734 -> [w2772]
          tunnel: w2731 -> [w2771] mode=indexing
          n1155 = call "App enquece.vi"("Priority Enquece"=TRUE, "command"=w2771, "queue in"=w2772) -> ("error out"=w2773:errorcluster, "Queue out"=w2774:refnum<queue>)  [unwired: 7 in]
        }
        n1156 = Merge Errors(w2739) -> (w2730:errorcluster)
        n1157 = Build Array("Test DRV 25", "Test DRV 26", "Test DRV 27", "Test DRV 28", "Test DRV 29", "Test DRV 30", "MEAS.requestAC") -> (w2745:string[])
        n1158 = Reverse 1D Array(array=w2745) -> (reversed array=w2746:string[])
        n1159 = for {
          tunnel: w2746 -> [w2780] mode=indexing
          tunnel: [w2779] -> w2738 mode=indexing
          shift-right: [w2778] -> w2729
          shift-left: w2740 -> [w2781]
          tunnel: w2730 -> [w2777]
          n1160 = call "App enquece.vi"("Priority Enquece"=TRUE, "error in (no error)"=w2777, "command"=w2780, "queue in"=w2781) -> ("error out"=w2779:errorcluster, "Queue out"=w2778:refnum<queue>)  [unwired: 6 in]
        }
        n1161 = Initialize Array(TRUE, 6 ("dimension size")) -> (w2757:bool[])
        n1162 = Merge Errors(w2738) -> (w2737:errorcluster)
        n1163 = To Variant(anything=T5."mux10_1_channel5" ("mux10_1(x6)_encode")) -> (Variant=w2766:variant)
        n1164 = To Variant(anything=T6."demux1_10_channel5" ("demux1_10(x6)_encode")) -> (Variant=w2762:variant)
        n1165 = To Variant(anything=w2757) -> (Variant=w2756:variant)
        n1166 = Bundle By Name(cluster=w2754, "command"="MEAS.mux10-1", "command data"=w2766) -> (w2761:T11)
        n1167 = Bundle By Name(cluster=w2754, "command"="MEAS.demux1-10", "command data"=w2762) -> (w2760:T11)
        n1168 = Bundle By Name(cluster=w2754, "command"="MEAS.eMIC", "command data"=w2756) -> (w2755:T11)
        n1169 = Build Array(w2761, w2760, w2755) -> (w2736:T11[])
        n1170 = Reverse 1D Array(array=w2736) -> (reversed array=w2735:T11[])
        n1171 = for {
          tunnel: w2735 -> [w2793] mode=indexing
          tunnel: [w2790] -> w2747 mode=indexing
          tunnel: w2737 -> [w2789]
          tunnel: w2729 -> [w2787]
          n1172 = Unbundle By Name(w2793) -> ("command"=w2792:string, "command data"=w2791:variant)
          n1173 = call "App enquece.vi"("Priority Enquece"=TRUE, "error in (no error)"=w2789, "command data"=w2791, "command"=w2792, "queue in"=w2787) -> ("error out"=w2790:errorcluster)  [unwired: 5 in, 1 out]
        }
        n1174 = Merge Errors(w2750, w2747) -> (w2751:errorcluster)
      }
      frame "Test Channel 6" {
        w2824 = 6  # DUT channel (1-11)
        w2825 = T11 {"command"="", "command data"=variant} ("element")
        n1175 = disable-structure shown="LOGGING==TRUE" {
          disable-tunnel: w2819 -> [w2854 _]
          frame condition #0 (active) {
            n1176 = Empty String/Path?(string/path=w2854) -> (empty?=w2857:bool)
            n1177 = Select(t="Quece timeout", s=w2857, f=w2854) -> (s? t:f=w2853:string)
            n1178 = call "string log (SubVI).vi"("Enum"=enum16{"Init", "Log", "Read"}."Log", "state Name"=w2853) -> ()  [unwired: 8 in, 2 out]
          }
          frame condition #1 {
          }
        }
        n1179 = Build Array("Apps.UI Update", "MEAS.AllRelaysOFF2", "Apps.WaitForEvent") -> (w2801:string[])
        n1180 = for {
          tunnel: [w2844] -> w2809 mode=indexing
          shift-right: [w2845] -> w2811
          shift-left: w2804 -> [w2843]
          tunnel: w2801 -> [w2842] mode=indexing
          n1181 = call "App enquece.vi"("Priority Enquece"=TRUE, "command"=w2842, "queue in"=w2843) -> ("error out"=w2844:errorcluster, "Queue out"=w2845:refnum<queue>)  [unwired: 7 in]
        }
        n1182 = Merge Errors(w2809) -> (w2800:errorcluster)
        n1183 = Build Array("Test DRV 31", "Test DRV 32", "Test DRV 33", "Test DRV 34", "Test DRV 35", "Test DRV 36", "MEAS.requestAC") -> (w2816:string[])
        n1184 = Reverse 1D Array(array=w2816) -> (reversed array=w2817:string[])
        n1185 = for {
          tunnel: w2817 -> [w2851] mode=indexing
          tunnel: [w2850] -> w2808 mode=indexing
          shift-right: [w2849] -> w2810
          shift-left: w2811 -> [w2852]
          tunnel: w2800 -> [w2848]
          n1186 = call "App enquece.vi"("Priority Enquece"=TRUE, "error in (no error)"=w2848, "command"=w2851, "queue in"=w2852) -> ("error out"=w2850:errorcluster, "Queue out"=w2849:refnum<queue>)  [unwired: 6 in]
        }
        n1187 = Initialize Array(TRUE, 6 ("dimension size")) -> (w2828:bool[])
        n1188 = Merge Errors(w2808) -> (w2807:errorcluster)
        n1189 = To Variant(anything=T5."mux10_1_channel6" ("mux10_1(x6)_encode")) -> (Variant=w2837:variant)
        n1190 = To Variant(anything=T6."demux1_10_channel6" ("demux1_10(x6)_encode")) -> (Variant=w2833:variant)
        n1191 = To Variant(anything=w2828) -> (Variant=w2827:variant)
        n1192 = Bundle By Name(cluster=w2825, "command"="MEAS.mux10-1", "command data"=w2837) -> (w2832:T11)
        n1193 = Bundle By Name(cluster=w2825, "command"="MEAS.demux1-10", "command data"=w2833) -> (w2831:T11)
        n1194 = Bundle By Name(cluster=w2825, "command"="MEAS.eMIC", "command data"=w2827) -> (w2826:T11)
        n1195 = Build Array(w2832, w2831, w2826) -> (w2806:T11[])
        n1196 = Reverse 1D Array(array=w2806) -> (reversed array=w2805:T11[])
        n1197 = for {
          tunnel: w2805 -> [w2863] mode=indexing
          tunnel: [w2860] -> w2818 mode=indexing
          tunnel: w2807 -> [w2859]
          tunnel: w2810 -> [w2864]
          n1198 = Unbundle By Name(w2863) -> ("command"=w2862:string, "command data"=w2861:variant)
          n1199 = call "App enquece.vi"("Priority Enquece"=TRUE, "error in (no error)"=w2859, "command data"=w2861, "command"=w2862, "queue in"=w2864) -> ("error out"=w2860:errorcluster)  [unwired: 5 in, 1 out]
        }
        n1200 = Merge Errors(w2821, w2818) -> (w2822:errorcluster)
      }
      frame "Test Channel 7" {
        w2895 = 7  # DUT channel (1-11)
        w2896 = T11 {"command"="", "command data"=variant} ("element")
        n1201 = disable-structure shown="LOGGING==TRUE" {
          disable-tunnel: w2890 -> [w2925 _]
          frame condition #0 (active) {
            n1202 = Empty String/Path?(string/path=w2925) -> (empty?=w2928:bool)
            n1203 = Select(t="Quece timeout", s=w2928, f=w2925) -> (s? t:f=w2924:string)
            n1204 = call "string log (SubVI).vi"("Enum"=enum16{"Init", "Log", "Read"}."Log", "state Name"=w2924) -> ()  [unwired: 8 in, 2 out]
          }
          frame condition #1 {
          }
        }
        n1205 = Build Array("Apps.UI Update", "MEAS.AllRelaysOFF2", "Apps.WaitForEvent") -> (w2874:string[])
        n1206 = for {
          tunnel: [w2915] -> w2881 mode=indexing
          shift-right: [w2916] -> w2882
          shift-left: w2877 -> [w2914]
          tunnel: w2874 -> [w2913] mode=indexing
          n1207 = call "App enquece.vi"("Priority Enquece"=TRUE, "command"=w2913, "queue in"=w2914) -> ("error out"=w2915:errorcluster, "Queue out"=w2916:refnum<queue>)  [unwired: 7 in]
        }
        n1208 = Merge Errors(w2881) -> (w2873:errorcluster)
        n1209 = Build Array("Test DRV 37", "Test DRV 38", "Test DRV 39", "Test DRV 40", "Test DRV 41", "Test DRV 42", "MEAS.requestAC") -> (w2887:string[])
        n1210 = Reverse 1D Array(array=w2887) -> (reversed array=w2888:string[])
        n1211 = for {
          tunnel: w2888 -> [w2922] mode=indexing
          tunnel: [w2921] -> w2880 mode=indexing
          shift-right: [w2920] -> w2872
          shift-left: w2882 -> [w2923]
          tunnel: w2873 -> [w2919]
          n1212 = call "App enquece.vi"("Priority Enquece"=TRUE, "error in (no error)"=w2919, "command"=w2922, "queue in"=w2923) -> ("error out"=w2921:errorcluster, "Queue out"=w2920:refnum<queue>)  [unwired: 6 in]
        }
        n1213 = Merge Errors(w2880) -> (w2879:errorcluster)
        n1214 = Initialize Array(TRUE, 6 ("dimension size")) -> (w2899:bool[])
        n1215 = To Variant(anything=w2899) -> (Variant=w2898:variant)
        n1216 = To Variant(anything=T5."mux10_1_channel7" ("mux10_1(x6)_encode")) -> (Variant=w2908:variant)
        n1217 = To Variant(anything=T6."demux1_10_channel7" ("demux1_10(x6)_encode")) -> (Variant=w2904:variant)
        n1218 = Bundle By Name(cluster=w2896, "command"="MEAS.mux10-1", "command data"=w2908) -> (w2903:T11)
        n1219 = Bundle By Name(cluster=w2896, "command"="MEAS.demux1-10", "command data"=w2904) -> (w2902:T11)
        n1220 = Bundle By Name(cluster=w2896, "command"="MEAS.eMIC", "command data"=w2898) -> (w2897:T11)
        n1221 = Build Array(w2903, w2902, w2897) -> (w2878:T11[])
        n1222 = Reverse 1D Array(array=w2878) -> (reversed array=w2871:T11[])
        n1223 = for {
          tunnel: w2871 -> [w2935] mode=indexing
          tunnel: [w2932] -> w2889 mode=indexing
